vi "DoorNeedingSpellDoor.vi"(8 "error in (no error)":errorcluster, 10 "Room 2":refnum<class "Room.lvclass">, 11 "Room 1":refnum<class "Room.lvclass">) -> (0 "error out":errorcluster, 3 "DoorNeedingSpell":refnum<class "DoorNeedingSpell.lvclass">)   [LabVIEW 2020, in "DoorNeedingSpell.lvclass"]
uses:
  DoorNeedingSpell.lvclass
  Room/Room.lvclass
  Room/Room.lvclass/Room.ctl
  Room/Property/roomNumber/Read roomNumber.vi
  MazeSite/MazeSite.lvclass
  Support/Class/ConsoleOutput.lvclass
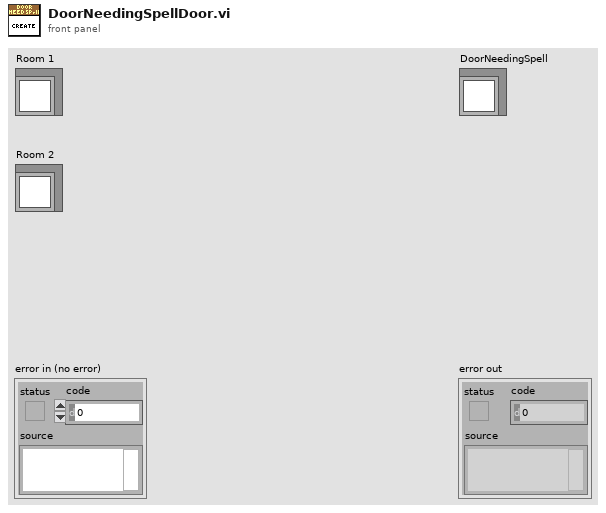
[diagram p1: front panel]
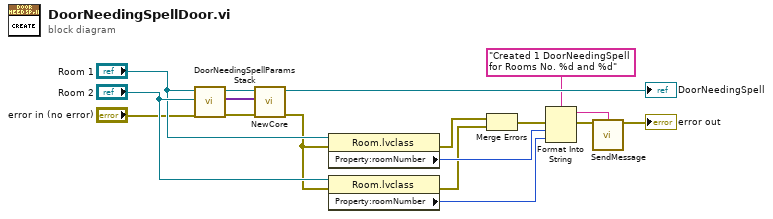
[diagram p0: block diagram]
diagram:
  n1 = call "DoorNeedingSpellParamsStack.vi"("error in (no error)"="error in (no error)", "room2"="Room 2", "room1"="Room 1") -> ("error out"=w17:errorcluster, "HierarchyParams"=w16:variant[], "DoorNeedingSpell"=w15:refnum<class "DoorNeedingSpell.lvclass">)  [unwired: 6 in]
  n2 = call-dynamic "NewCore.vi"("error in (no error)"=w17, "ParamsArray"=w16, "DoorNeedingSpell"=w15) -> ("error out"=w2:errorcluster, "DoorNeedingSpell"=→"DoorNeedingSpell":refnum<class "DoorNeedingSpell.lvclass">)  [unwired: 7 in]
  n3 = property class="Room.lvclass"(reference="Room 1", error in=w2) -> (error out=w5:errorcluster, "Property:roomNumber"=w8:i32)  [unwired: 1 out]
  n4 = property class="Room.lvclass"(reference="Room 2", error in=w2) -> (error out=w4:errorcluster, "Property:roomNumber"=w7:i32)  [unwired: 1 out]
  n5 = Merge Errors(w5, w4) -> (w3:errorcluster)
  n6 = Format Into String(format string="Created 1 DoorNeedingSpell for Rooms No. %d and %d" ("Message"), error in=w3, w8, w7) -> (resulting string=w13:string, error out=w12:errorcluster)  [unwired: 1 in]
  n7 = call "SendMessage.vi"("Message"=w13, "error in (no error)"=w12) -> ("error out"=→"error out":errorcluster)  [unwired: 13 in]
